vi "Get Plugin Pointers.vi"(8 "error in (no error)":errorcluster, 10 "plugin index":i32, 11 "Framework Status in":refnum<class "Framework Status.lvclass">) -> (0 "error out":errorcluster, 1 "group status pointers":refnum<class "Status Pointer.lvclass">[](array[class]), 2 "plugin status pointer":refnum<class "Status Pointer.lvclass">, 3 "Framework Status out":refnum<class "Framework Status.lvclass">)   [LabVIEW 2017, in "DSF Core.lvlib" / "Framework Status.lvclass"]
uses:
  Framework Status.lvclass
  Status/Status Pointer.lvclass
  Framework Status.lvclass/Framework Status.ctl
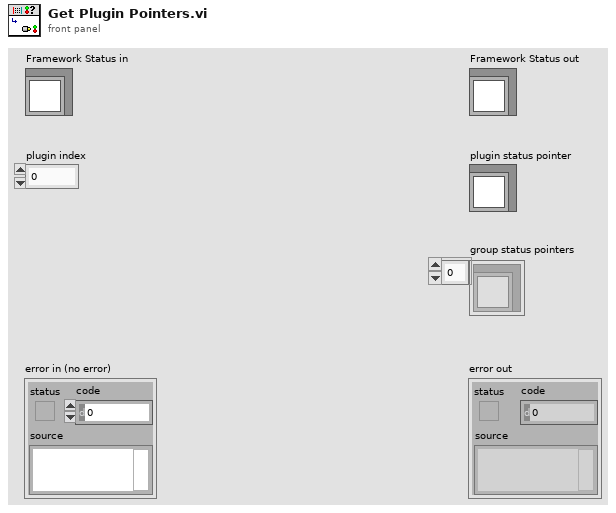
[diagram p1: front panel]
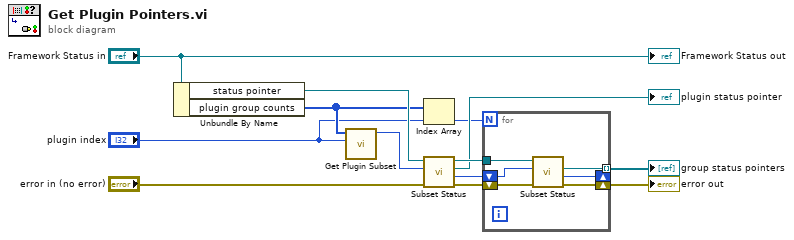
[diagram p0: block diagram]
diagram:
  n1 = Unbundle By Name("Framework Status in") -> ("status pointer"=w10:refnum<class "Status Pointer.lvclass">, "plugin group counts"=w9:u8[])
  n2 = call "Get Plugin Subset.vi"("plugin index"="plugin index", "plugin group counts"=w9) -> ("index"=w12:i32)  [unwired: 8 in, 1 out]
  n3 = Index Array(array=w9, index="plugin index") -> (element=w2:u8)
  n4 = call "Subset Status.vi"("error in (no error)"="error in (no error)", "index"=w12, "status pointer in"=w10) -> ("error out"=w7:errorcluster, "index + count"=w6:u64, "subset status pointer"=→"plugin status pointer":refnum<class "Status Pointer.lvclass">, "status pointer out"=w5:refnum<class "Status Pointer.lvclass">)  [unwired: 5 in]
  n5 = for {
    N: w2 -> [_]
    shift-right: [w18] -> w1
    shift-left: w7 -> [w19]
    shift-right: [w16] -> _
    shift-left: w6 -> [w17]
    tunnel: w5 -> [w15]
    tunnel: [w14] -> w3 mode=indexing
    n6 = call "Subset Status.vi"("error in (no error)"=w19, "index"=w17, "status pointer in"=w15) -> ("error out"=w18:errorcluster, "index + count"=w16:u64, "subset status pointer"=w14:refnum<class "Status Pointer.lvclass">)  [unwired: 5 in, 1 out]
  }
  "error out" <- w1
  "group status pointers" <- w3
  "Framework Status out" <- "Framework Status in"
